vi "Set Waveform Graph Plot Style.vi"(8 "Error In":errorcluster, 9 "Plot Index (0)":i32, 10 "Plot Style":T1, 11 "Graph in":refnum<vi>) -> (0 "Error Out":errorcluster)   [LabVIEW 2019]
uses:
  Single Plot Style 2.ctl
  Plot Style Settings Step.ctl
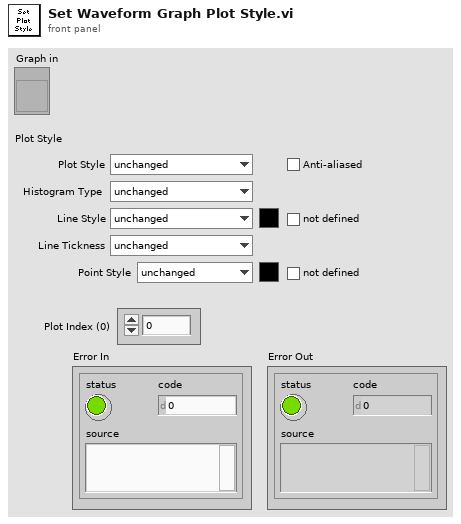
[diagram p1: front panel]
types:
  T1 = typedef "Single Plot Style 2.ctl" = cluster{"Plot Style":enum16{"unchanged", "Line", "Symbol", "Line + Symbol", "Histogram", "Histogram + Symbol"}, "Histogram Type":enum16{"unchanged", "Left Bound", "Center", "Right Bound"}, "Line Tickness":enum16{"unchanged", "Thin", "1 pixel", "2 pixel", "3 pixel", "4 pixel", "5 pixel"}, "Line Style":enum16{"unchanged", "Plain", "Long Dash", "Short Dash", "Long-Short Dash", "Long-Short-Short Dash"}, "Point Style":enum16{"unchanged", "None", "Empty Circle", "Filled Circle", "Thick Circle", "Dotted Circle", "Empty Square", "Filled Square", "Thick Square", "Dotted Square", "Small Filled Square", "Dot", "Cross", "Tiny Cross", "Large X", "Small x", "Diamond", "Small Empty Square"}, "Line Color":u32, "Line Color defined?":bool, "Point Color":u32, "Point Color defined?":bool, "Anti-aliased":bool}
  T2 = typedef "Plot Style Settings Step.ctl" = enum16{"Plot Type", "Line Style", "Line Thickness", "Line Color", "Point Style", "Point Color", "Aliasing"}
  T3 = enum16{"unchanged", "Line", "Symbol", "Line + Symbol", "Histogram", "Histogram + Symbol"}
  T4 = enum16{"unchanged", "Left Bound", "Center", "Right Bound"}
  T5 = enum16{"unchanged", "Plain", "Long Dash", "Short Dash", "Long-Short Dash", "Long-Short-Short Dash"}
  T6 = enum16{"unchanged", "Thin", "1 pixel", "2 pixel", "3 pixel", "4 pixel", "5 pixel"}
  T7 = enum16{"unchanged", "None", "Empty Circle", "Filled Circle", "Thick Circle", "Dotted Circle", "Empty Square", "Filled Square", "Thick Square", "Dotted Square", "Small Filled Square", "Dot", "Cross", "Tiny Cross", "Large X", "Small x", "Diamond", "Small Empty Square"}
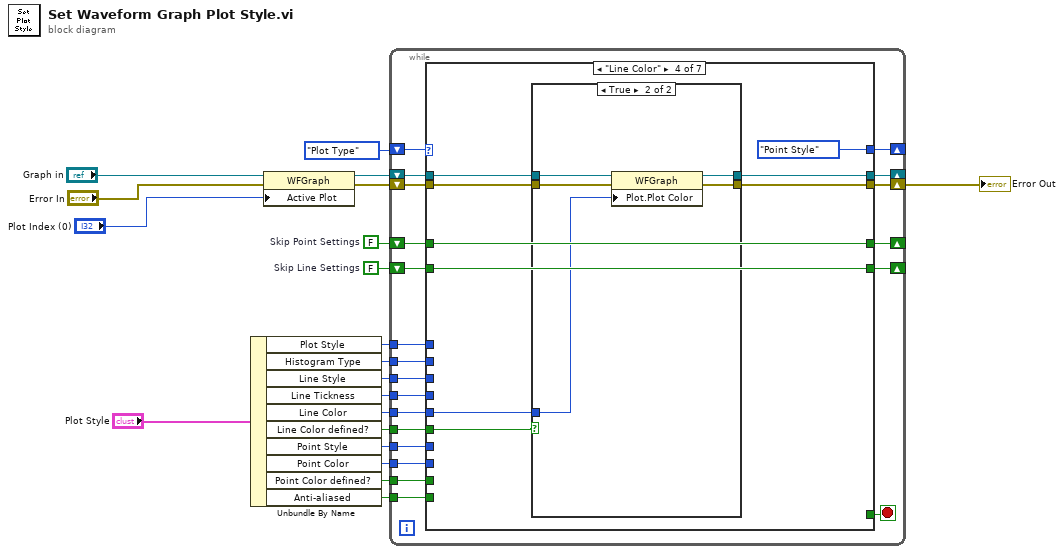
[diagram p0: block diagram]
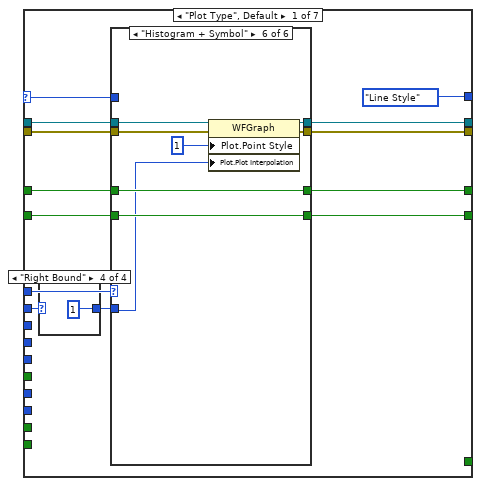
[diagram p2: hidden frame]
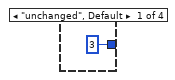
[diagram p3: hidden frame]
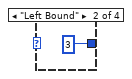
[diagram p4: hidden frame]
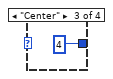
[diagram p5: hidden frame]
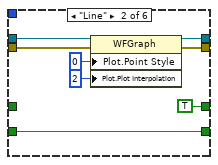
[diagram p7: hidden frame]
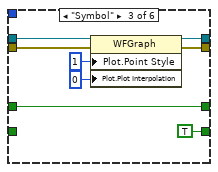
[diagram p8: hidden frame]
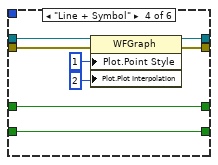
[diagram p9: hidden frame]
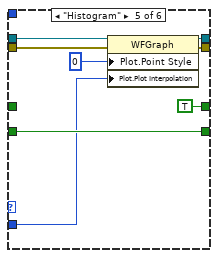
[diagram p10: hidden frame]
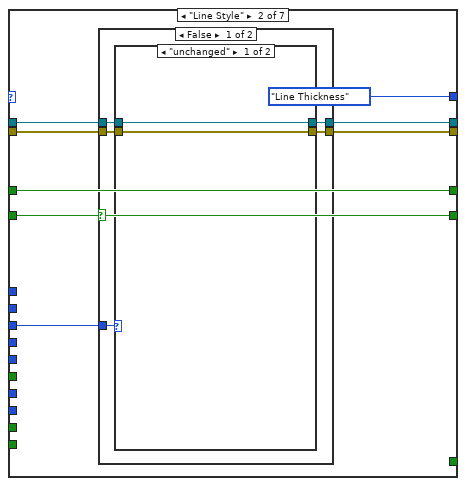
[diagram p11: hidden frame]
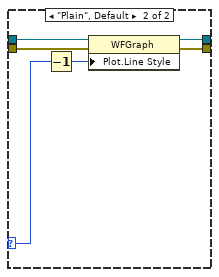
[diagram p12: hidden frame]
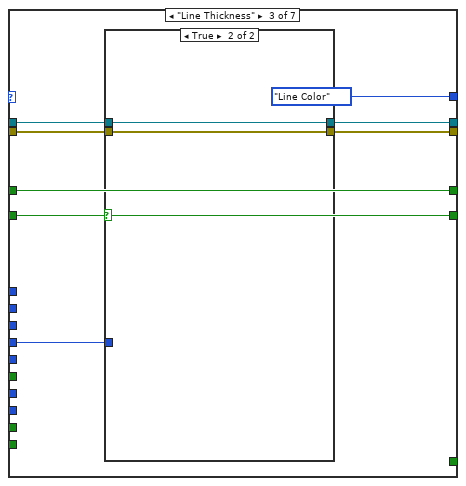
[diagram p14: hidden frame]
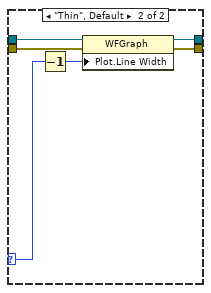
[diagram p16: hidden frame]
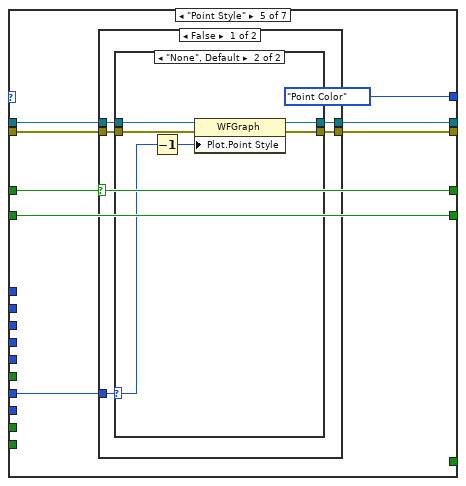
[diagram p18: hidden frame]
diagram:
  w1 = FALSE  # Skip Line Settings
  w2 = FALSE  # Skip Point Settings
  n1 = Unbundle By Name("Plot Style") -> ("Plot Style"=w15:T3, "Histogram Type"=w14:T4, "Line Style"=w10:T5, "Line Tickness"=w9:T6, "Line Color"=w8:u32, "Line Color defined?"=w7:bool, "Point Style"=w6:T7, "Point Color"=w4:u32, "Point Color defined?"=w5:bool, "Anti-aliased"=w3:bool)
  n2 = property class="WFGraph"(reference="Graph in", error in="Error In", "Active Plot"="Plot Index (0)") -> (reference out=w13:refnum<vi>, error out=w12:errorcluster)
  n3 = while {
    shift-right: [w36] -> _
    shift-left: Plot_Style_Settings_Step."Plot Type" ("Plot Style Step") -> [w41]
    tunnel: w15 -> [w40]
    tunnel: w14 -> [w39]
    shift-right: [w35] -> _
    shift-left: w13 -> [w38]
    shift-right: [w34] -> w11
    shift-left: w12 -> [w37]
    tunnel: w10 -> [w33]
    tunnel: w9 -> [w32]
    tunnel: w8 -> [w31]
    tunnel: w7 -> [w30]
    tunnel: w6 -> [w29]
    tunnel: w5 -> [w28]
    tunnel: w4 -> [w27]
    tunnel: w3 -> [w26]
    shift-right: [w23] -> _
    shift-left: w2 -> [w24]
    shift-right: [w21] -> _
    shift-left: w1 -> [w22]
    stop <- w25 stop-if-true
    n4 = case shown="\"Line Color\"" w41 {
      selector: w41 -> [w52 _ _ _ _ _ _]
      tunnel: w40 -> [w54 _ _ _ _ _ _]
      tunnel: w39 -> [w43 _ _ _ _ _ _]
      tunnel: w38 -> [w53 w109 w133 w157 w172 w196 w220]
      tunnel: w37 -> [w51 w107 w131 w155 w170 w194 w218]
      tunnel: [Plot_Style_Settings_Step."Line Style" ("Plot Style Step") Plot_Style_Settings_Step."Line Thickness" ("Plot Style Step") Plot_Style_Settings_Step."Line Color" ("Plot Style Step") Plot_Style_Settings_Step."Point Style" ("Plot Style Step") Plot_Style_Settings_Step."Point Color" ("Plot Style Step") Plot_Style_Settings_Step."Aliasing" ("Plot Style Step") Plot_Style_Settings_Step."Aliasing" ("Plot Style Step")] -> w36
      tunnel: [w49 w108 w132 w156 w171 w195 w219] -> w35
      tunnel: [w48 w106 w130 w154 w169 w193 w217] -> w34
      tunnel: w33 -> [_ w110 _ _ _ _ _]
      tunnel: w32 -> [_ _ w128 _ _ _ _]
      tunnel: w31 -> [_ _ _ w151 _ _ _]
      tunnel: w30 -> [_ _ _ w152 _ _ _]
      tunnel: w29 -> [_ _ _ _ w167 _ _]
      tunnel: w28 -> [_ _ _ _ _ w191 _]
      tunnel: w27 -> [_ _ _ _ _ w190 _]
      tunnel: w26 -> [_ _ _ _ _ _ w215]
      tunnel: [_ _ _ _ _ _ TRUE] -> w25
      tunnel: w24 -> [w47 w104 w127 w150 w166 w189 w213]
      tunnel: [w46 w104 w127 w150 w166 w189 w213] -> w23
      tunnel: w22 -> [w45 w103 w126 w149 w165 w188 w212]
      tunnel: [w44 w103 w126 w149 w165 w188 w212] -> w21
      frame "Plot Type", Default {
        n5 = case shown="\"Right Bound\"" w43 {
          tunnel: [u16 3 ("y") u16 3 ("y") u16 4 ("y") u16 1 ("y")] -> w42
          frame "unchanged", Default {
          }
          frame "Left Bound" {
          }
          frame "Center" {
          }
          frame "Right Bound" {
          }
        }
        n6 = case shown="\"Histogram + Symbol\"" w54 {
          tunnel: w42 -> [_ _ _ _ w87 w95]
          tunnel: w53 -> [w62 w70 w78 w86 w94 w102]
          tunnel: w52 -> [_ _ _ _ _ _]
          tunnel: w51 -> [w61 w68 w76 w84 w92 w100]
          tunnel: [w62 w69 w77 w85 w93 w101] -> w49
          tunnel: [w61 w67 w75 w83 w91 w99] -> w48
          tunnel: w47 -> [w60 _ w72 w81 _ w97]
          tunnel: [w60 TRUE ("Skip Point Settings") w72 w81 TRUE ("Skip Point Settings") w97] -> w46
          tunnel: w45 -> [w59 w64 _ w80 w89 w98]
          tunnel: [w59 w64 TRUE ("Skip Line Settings") w80 w89 w98] -> w44
          frame "unchanged", Default {
          }
          frame "Line" {
            n7 = property class="WFGraph"(reference=w70, error in=w68, "Plot.Point Style"=u8 0, "Plot.Plot Interpolation"=u8 2 ("Plot.Point Style")) -> (reference out=w69:refnum<vi>, error out=w67:errorcluster)
          }
          frame "Symbol" {
            n8 = property class="WFGraph"(reference=w78, error in=w76, "Plot.Point Style"=u8 1, "Plot.Plot Interpolation"=u8 0) -> (reference out=w77:refnum<vi>, error out=w75:errorcluster)
          }
          frame "Line + Symbol" {
            n9 = property class="WFGraph"(reference=w86, error in=w84, "Plot.Point Style"=u8 1, "Plot.Plot Interpolation"=u8 2) -> (reference out=w85:refnum<vi>, error out=w83:errorcluster)
          }
          frame "Histogram" {
            n10 = property class="WFGraph"(reference=w94, error in=w92, "Plot.Point Style"=u8 0, "Plot.Plot Interpolation"=w87) -> (reference out=w93:refnum<vi>, error out=w91:errorcluster)
          }
          frame "Histogram + Symbol" {
            n11 = property class="WFGraph"(reference=w102, error in=w100, "Plot.Point Style"=u8 1, "Plot.Plot Interpolation"=w95) -> (reference out=w101:refnum<vi>, error out=w99:errorcluster)
          }
        }
      }
      frame "Line Style" {
        n12 = case shown="False" w103 {
          tunnel: w110 -> [w115 _]
          tunnel: w109 -> [w114 w125]
          tunnel: [w113 w125] -> w108
          tunnel: w107 -> [w112 w124]
          tunnel: [w111 w124] -> w106
          frame False {
            n13 = case shown="\"unchanged\"" w115 {
              selector: w115 -> [_ w122]
              tunnel: w114 -> [w117 w123]
              tunnel: [w117 w121] -> w113
              tunnel: w112 -> [w116 w119]
              tunnel: [w116 w120] -> w111
              frame "unchanged" {
              }
              frame "Plain", Default {
                n14 = Decrement(x=w122) -> (x-1=w118:T5)
                n15 = property class="WFGraph"(reference=w123, error in=w119, "Plot.Line Style"=w118) -> (reference out=w121:refnum<vi>, error out=w120:errorcluster)
              }
            }
          }
          frame True {
          }
        }
      }
      frame "Line Thickness" {
        n16 = case shown="True" w126 {
          tunnel: w133 -> [w138 w148]
          tunnel: [w137 w148] -> w132
          tunnel: w131 -> [w136 w147]
          tunnel: [w135 w147] -> w130
          tunnel: w128 -> [w134 _]
          frame False {
            n17 = case shown="\"unchanged\"" w134 {
              selector: w134 -> [_ w145]
              tunnel: w138 -> [w140 w146]
              tunnel: [w140 w144] -> w137
              tunnel: w136 -> [w139 w142]
              tunnel: [w139 w143] -> w135
              frame "unchanged" {
              }
              frame "Thin", Default {
                n18 = Decrement(x=w145) -> (x-1=w141:T6)
                n19 = property class="WFGraph"(reference=w146, error in=w142, "Plot.Line Width"=w141) -> (reference out=w144:refnum<vi>, error out=w143:errorcluster)
              }
            }
          }
          frame True {
          }
        }
      }
      frame "Line Color" {
        n20 = case shown="True" w152 {
          tunnel: w157 -> [w159 w164]
          tunnel: [w159 w163] -> w156
          tunnel: w155 -> [w158 w161]
          tunnel: [w158 w162] -> w154
          tunnel: w151 -> [_ w160]
          frame False {
          }
          frame True {
            n21 = property class="WFGraph"(reference=w164, error in=w161, "Plot.Plot Color"=w160) -> (reference out=w163:refnum<vi>, error out=w162:errorcluster)
          }
        }
      }
      frame "Point Style" {
        n22 = case shown="False" w166 {
          tunnel: w172 -> [w177 w187]
          tunnel: [w176 w187] -> w171
          tunnel: w170 -> [w175 w186]
          tunnel: [w174 w186] -> w169
          tunnel: w167 -> [w173 _]
          frame False {
            n23 = case shown="\"None\", Default" w173 {
              selector: w173 -> [_ w184]
              tunnel: w177 -> [w179 w185]
              tunnel: [w179 w183] -> w176
              tunnel: w175 -> [w178 w181]
              tunnel: [w178 w182] -> w174
              frame "unchanged" {
              }
              frame "None", Default {
                n24 = Decrement(x=w184) -> (x-1=w180:T7)
                n25 = property class="WFGraph"(reference=w185, error in=w181, "Plot.Point Style"=w180) -> (reference out=w183:refnum<vi>, error out=w182:errorcluster)
              }
            }
          }
          frame True {
          }
        }
      }
      frame "Point Color" {
        n26 = case shown="False" w189 {
          tunnel: w196 -> [w202 w211]
          tunnel: [w201 w211] -> w195
          tunnel: w194 -> [w200 w210]
          tunnel: [w199 w210] -> w193
          tunnel: w191 -> [w198 _]
          tunnel: w190 -> [w197 _]
          frame False {
            n27 = case shown="True" w198 {
              tunnel: w202 -> [w204 w209]
              tunnel: [w204 w208] -> w201
              tunnel: w200 -> [w203 w206]
              tunnel: [w203 w207] -> w199
              tunnel: w197 -> [_ w205]
              frame False {
              }
              frame True {
                n28 = property class="WFGraph"(reference=w209, error in=w206, "Plot.Fill/Pt. Color"=w205) -> (reference out=w208:refnum<vi>, error out=w207:errorcluster)
              }
            }
          }
          frame True {
          }
        }
      }
      frame "Aliasing" {
        n29 = property class="WFGraph"(reference=w220, error in=w218, "Plot.Anti-aliased"=w215) -> (reference out=w219:refnum<vi>, error out=w217:errorcluster)
      }
    }
  }
  "Error Out" <- w11
